vi "Ödev.vi"(9 "Outpt ( Trig ) Pin":u8, 10 "Ýnput ( Echo ) Pin":u8) -> (1 "Santimetre":dbl)   [LabVIEW 2017]
uses:
  <vilib>/MakerHub/LINX/Private/Device/Type Defs/Stimulus Pulse.ctl
  <vilib>/MakerHub/LINX/Private/Device/Type Defs/Pulse Polarity.ctl
  <vilib>/MakerHub/LINX/Public/Utilities/Open Serial.vi
  <vilib>/MakerHub/LINX/LMH-LINX.lvlib
  <vilib>/MakerHub/LINX/Private/Device/Device.lvlib
panel:
  in  "Durdur":bool
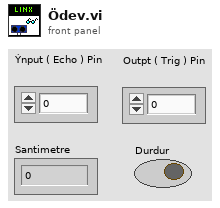
[diagram p1: front panel]
types:
  T1 = typedef "LMH-LINX.lvlib/LINX Ref.ctl" = cluster{"IO":T2, "Interface":T3, "LINX Device Config":T4}
  T2 = typedef "LMH-LINX.lvlib/Platform.ctl" = enum16{"Remote", "Local"}
  T3 = typedef "LMH-LINX.lvlib/Interface.ctl" = enum16{"Serial", "TCP"}
  T4 = typedef "LMH-LINX.lvlib/Device.lvlib/LINX Device Config.ctl" = cluster{"Interface":T3, "COM Port":refnum<visa-resource-name>, "TCP Configuration":T5, "Device Family":u8, "Device ID":u8, "Device Name":string, "TCP Ref":refnum<k5>, "Channels":T6}
  T5 = typedef "LMH-LINX.lvlib/Device.lvlib/TCP Config.ctl" = cluster{"IP Address":string, "Port":u16}
  T6 = typedef "LMH-LINX.lvlib/Channels.ctl" = cluster{"DI":u8[], "DO":u8[], "AI":u8[], "AO":u8[], "PWM":u8[], "QE":u8[], "UART":u8[], "I2C 2":u8[], "SPI":u8[], "CAN":u8[], "Servo":u8[], "AI Ref (V)":dbl, "AI Resolution (Bits)":u8, "AO Ref (V)":dbl, "AO Resolution (Bits)":u8}
  T7 = typedef "LMH-LINX.lvlib/Device.lvlib/Pulse Polarity.ctl" = enum8{"Active Low", "Active High"}
  T8 = typedef "LMH-LINX.lvlib/Device.lvlib/Stimulus Pulse.ctl" = enum16{"None", "Active Low", "Active High"}
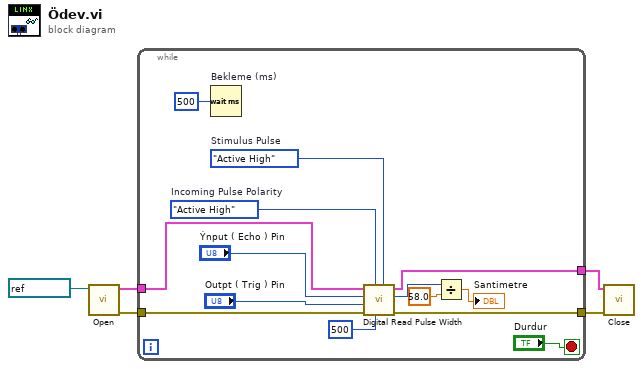
[diagram p0: block diagram]
diagram:
  n1 = call-poly <vilib>:"Open.vi"("Serial Port"=refnum<visa-resource-name> "COM6") -> ("Error Out"=w2:errorcluster, "LINX Resource"=w5:T1)  [unwired: 8 in, 1 out]
  n2 = while {
    tunnel: w5 -> [w11]
    tunnel: [w10] -> w4
    tunnel: [w9] -> w3
    tunnel: w2 -> [w8]
    stop <- "Durdur" stop-if-true
    w12 = Pulse_Polarity."Active High"  # Incoming Pulse Polarity
    w13 = Stimulus_Pulse."Active High"  # Stimulus Pulse
    n3 = Wait (ms) "Bekleme (ms)"(milliseconds to wait=u32 500) -> ()  [unwired: 1 out]
    n4 = call <vilib>:"Digital Read Pulse Width.vi"("Stimulus Pulse (Active High)"=w13, "Timeout  (250 mS)"=u32 500, "Incoming Pulse Polarity (Active High)"=w12, "Error In"=w8, "DO Channel"="Outpt ( Trig ) Pin", "DI Channel"="Ýnput ( Echo ) Pin", "LINX Resource"=w11) -> ("Error Out"=w9:errorcluster, "Pulse Width (uS)"=w16:u32, "LINX Resource"=w10:T1)  [unwired: 2 in]
    n5 = Divide(x=w16, y=58.0) -> (x/y=→"Santimetre":dbl)
  }
  n6 = call <vilib>:"Close.vi"("Error In"=w3, "LINX Resource"=w4) -> ()  [unwired: 9 in, 1 out]
